vi "Create Filename.vi"(10 "lab?":string, 11 "Array":string[](array[string])) -> (3 "Filename Output":string)   [LabVIEW 2018]
uses:
  Utility/Save File/Save File.lvlib
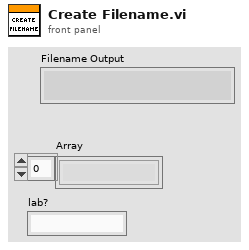
[diagram p1: front panel]
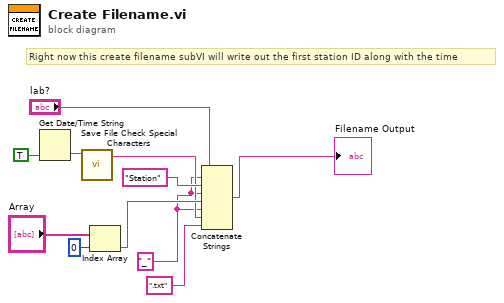
[diagram p0: block diagram]
diagram:
  w2 = "_" ("string")
  # "Right now this create filename subVI will write out the first station ID along with the time"
  n1 = Get Date/Time String(want seconds? (F)=TRUE) -> (time string=w11:string)  [unwired: 2 in, 1 out]
  n2 = call "Save File Check Special Characters.vi"("Filename"=w11) -> ("Filename Output"=w4:string)  [unwired: 9 in, 1 out]
  n3 = Index Array(array="Array", index=0) -> (element=w5:string)
  n4 = Concatenate Strings("lab?", w2, "Station" ("string"), w2, w5, w2, w4, ".txt" ("string")) -> (→"Filename Output":string)
